vi "Operate on single VI.vi"(8 "error in (no error)":errorcluster, 10 "LVClass.Open in":refnum<vi>, 11 "Application in":refnum<vi>) -> (0 "error out":errorcluster, 1 "Array":string[][](array[string]), 2 "LVClass.Open out":refnum<vi>, 3 "Application out":refnum<vi>)   [LabVIEW 2020]
uses:
  <userlib>/_OpenG.lib/appcontrol/appcontrol.llb/openg_application_control.lvlib
  <userlib>/_OpenG.lib/appcontrol/appcontrol.llb/Close Generic Object Refnum (Array)__ogtk.vi
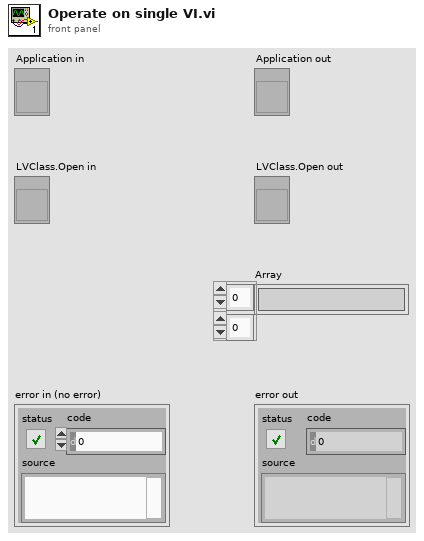
[diagram p1: front panel]
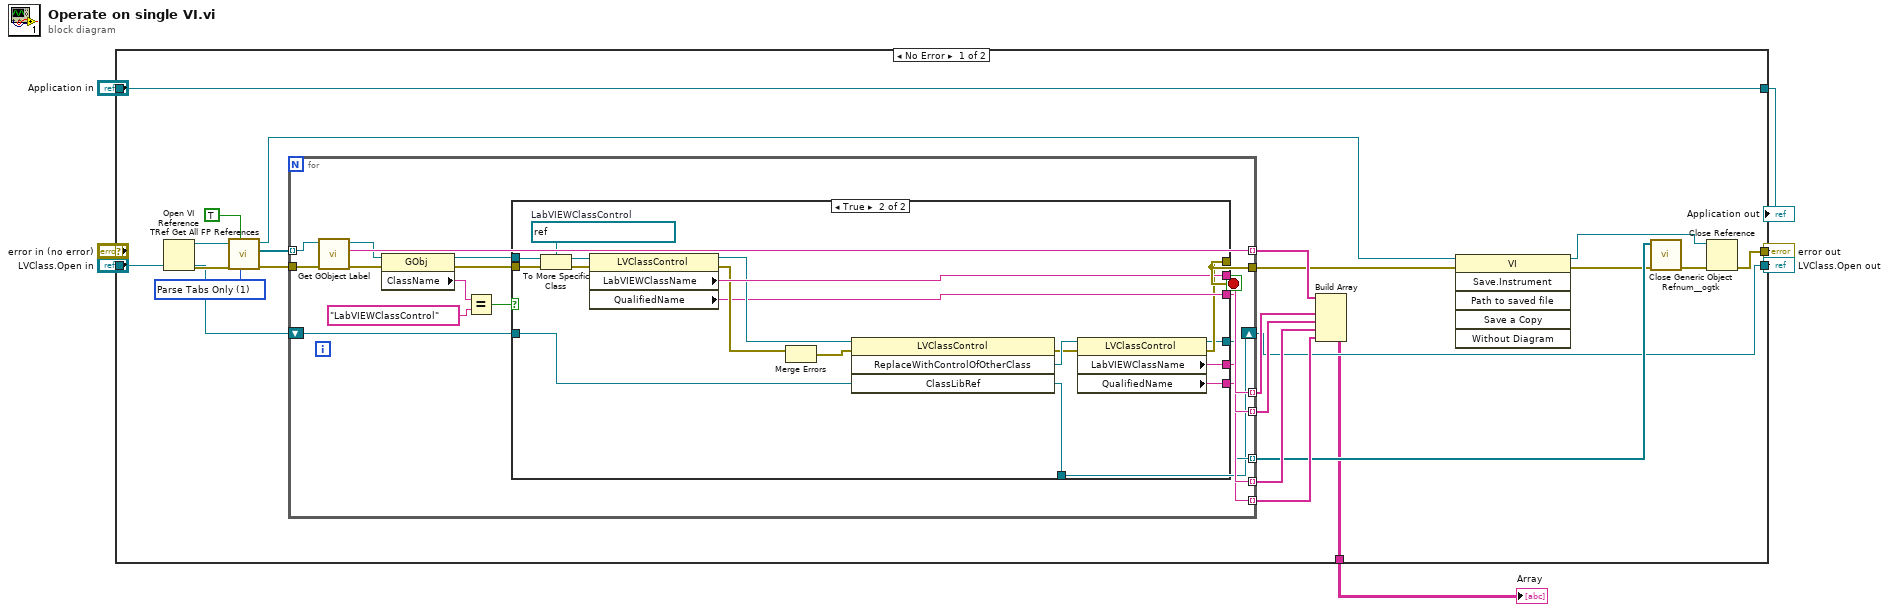
[diagram p0: block diagram]
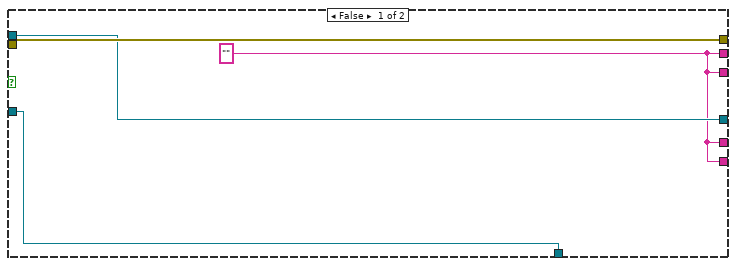
[diagram p2: hidden frame]
diagram:
  n1 = case shown="No Error" "error in (no error)" {
    selector: "error in (no error)" -> [_ w71]
    tunnel: [w23 w71] -> w1
    tunnel: "LVClass.Open in" -> [w11 w70]
    tunnel: "Application in" -> [w10 w72]
    tunnel: [w10 w72] -> w5
    tunnel: [w9 w70] -> w6
    tunnel: [w8 _] -> w7
    frame No Error {
      w26 = u16 1 items=["Parse All", "Parse Tabs Only"] ("Parsing Rule")
      n2 = Open VI Reference() -> (vi reference=w28:refnum<vi>, error out=w27:errorcluster)  [unwired: 6 in]
      n3 = call <vilib>:"TRef Get All FP References.vi"("Parsing Rule"=w26, "Ignore Decorations?"=TRUE, "error in (no error)"=w27, "VI Refnum"=w28) -> ("error out"=w24:errorcluster, "All FP Objects"=w25:refnum<vi>[], "dup VI Refnum"=w15:refnum<vi>)  [unwired: 3 in, 2 out]
      n4 = for {
        tunnel: w25 -> [w46] mode=indexing
        tunnel: w24 -> [w47]
        tunnel: [w45] -> w22 mode=indexing
        tunnel: [w37] -> w13
        tunnel: [w36] -> w21 mode=indexing
        tunnel: [w35] -> w20 mode=indexing
        tunnel: [w34] -> w19 mode=indexing
        tunnel: [w33] -> w18 mode=indexing
        tunnel: [w32] -> w17 mode=indexing
        shift-right: [w30] -> w9
        shift-left: w11 -> [w31]
        stop <- w37 stop-if-true
        n5 = call <vilib>:"Get GObject Label.vi"("error in (no error)"=w47, "GObject"=w46) -> ("error out"=w43:errorcluster, "Object Label"=w45:string, "dup GObject"=w44:refnum<vi>)  [unwired: 5 in, 2 out]
        n6 = property class="GObj"(reference=w44, error in=w43) -> (reference out=w38:refnum<vi>, error out=w39:errorcluster, "ClassName"=w42:string)
        n7 = Equal?(x=w42, y="LabVIEWClassControl") -> (x = y?=w40:bool)
        n8 = case shown="True" w40 {
          tunnel: w38 -> [w50 w69]
          tunnel: w39 -> [w51 w67]
          tunnel: [w49 w64] -> w36
          tunnel: [w49 w61] -> w35
          tunnel: [w51 w55] -> w37
          tunnel: [w49 w57] -> w34
          tunnel: [w49 w56] -> w33
          tunnel: [w50 w54] -> w32
          tunnel: w31 -> [w48 w53]
          tunnel: [w48 w52] -> w30
          frame False {
            w49 = "" ("LabVIEWClassName")
          }
          frame True {
            w68 = refnum<vi> refnum  # LabVIEWClassControl
            n9 = To More Specific Class(target class=w68, reference=w69, error in=w67) -> (specific class reference=w66:refnum<vi>, error out=w65:errorcluster)
            n10 = property class="LVClassControl"(reference=w66, error in=w65) -> (reference out=w63:refnum<vi>, error out=w62:errorcluster, "LabVIEWClassName"=w64:string, "QualifiedName"=w61:string)
            n11 = Merge Errors(w62) -> (w60:errorcluster)  [unwired: 1 in]
            n12 = invoke class="LVClassControl" method="ReplaceWithControlOfOtherClass"(reference=w63, error in=w60, "ClassLibRef"=w53) -> (error out=w58:errorcluster, "ReplaceWithControlOfOtherClass"=w59:refnum<vi>, "ClassLibRef"=w52:refnum<vi>)  [unwired: 1 in, 1 out]
            n13 = property class="LVClassControl"(reference=w59, error in=w58) -> (reference out=w54:refnum<vi>, error out=w55:errorcluster, "LabVIEWClassName"=w57:string, "QualifiedName"=w56:string)
          }
        }
      }
      n14 = Build Array(w22, w21, w20, w19, w18) -> (w8:string[][])  [unwired: 1 in]
      n15 = invoke class="VI" method="Save.Instrument"(reference=w15, error in=w13) -> (reference out=w14:refnum<vi>, error out=w12:errorcluster)  [unwired: 4 in, 4 out]
      n16 = call-poly <userlib>:"Close Generic Object Refnum__ogtk.vi"("error in (no error)"=w12, "Gen Refnum Array"=w17) -> ("error out"=w16:errorcluster)  [unwired: 9 in]
      n17 = Close Reference(reference=w14, error in (no error)=w16) -> (error out=w23:errorcluster)
    }
    frame Error {
    }
  }
  "Array" <- w7
  "LVClass.Open out" <- w6
  "Application out" <- w5
  "error out" <- w1
